vi "nanocal -- nuclear schottky fit V4.vi"() -> ()   [LabVIEW 2020]
uses:
  filename-pattern.ctl
  show-win- control.ctl
  cursor winow.ctl
  nanocal_data_read_format.ctl
  nanocal-goodness-weighting-strategy.ctl
  <vilib>/gmath/NumericalOptimization/stopping criteria.ctl
  3-lorentzian-parameters.ctl
  3-lorentzian-heat-response action.ctl
  nameformattingitem.ctl
  nanocal_side_selector.ctl
  filename-action.ctl
  cursor window action.ctl
  cursor action.ctl
  publisher action.ctl
  mathematica string map action.ctl
  array action.ctl
  cursor sate.ctl
  <vilib>/gmath/NumericalOptimization/objective function data.ctl
  3-lorentzian-parameters -- action.ctl
  <vilib>/Utility/miscctls.llb/LVMapReplaceAction.ctl
  file -- read-write control.ctl
  array -- freq-voltage transformations action.ctl
  nanocal_raw_file_manage_action_V1.ctl
  KM_file -- read-write control.ctl
  2Dwindow.ctl
  replace cursor action stack.vi
  Q -- range multiplier -- real -- V2.vi
  Q - not nan and gtr than zero - Real.vi
  Q - not nan -- real.vi
  Q -- check range -- i -- real.vi
  array - smart min max.vi
  3-lorentzian-heat-response -- analytic derivatives -- grad and curvature -- V4.vi
  <vilib>/Analysis/baseanly.llb/A x B.vi
  <vilib>/Analysis/baseanly.llb/Real A x B.vi
  <vilib>/Analysis/_algsub.llb/Matrix Norm.vi
  <vilib>/Analysis/_algsub.llb/Real Matrix Norm.vi
  3-lorentzian-heat-response -- V4.vi/142dd4c5-f9ed-c64b-bc14-a88e3e2c450a.vi
  array -- freq-voltage transformations.vi/05c44075-957c-bc42-b6fa-2799d0bc0485.vi
  tale of three indices.vi
  filter -- window span logic.vi
  linear interp iiii- complex - z-omega - divide.vi
  linear interpolation iiii- complex.vi
  containing bix.vi
  3-lorentzian-heat-response.vi/142dd4c5-f9ed-c64b-bc14-a88e3e2c450a.vi
  <vilib>/Array/Sort 2D Array - Pop Stack.vi
  <vilib>/Array/Sort 2D Array - Push Stack.vi
  array -- freq-voltage transformations.vi/05c44075-957c-bc42-b6fa-2799d0bc0485.vi/5dd0d2be-718e-c148-b8fa-e083cdba2843.vi
  array -- freq-voltage transformations.vi/05c44075-957c-bc42-b6fa-2799d0bc0485.vi/095795a0-771d-c341-9fed-d90d2e44c51c.vi
  command stack.vi
  tale of three indices -- check state.vi
  Q -- check range -- i -- integer.vi
  linear interp iiii- complex - z-omega.vi
  line -- complex.vi
  Q - not nan -- integer.vi
  <vilib>/Analysis/baseanly.llb/Complex A x B.vi
  <vilib>/Analysis/polynomials.llb/Multiply Polynomials.vi
  <vilib>/Analysis/polynomials.llb/Multiply Polynomials (DBL).vi
  <vilib>/Analysis/polynomials.llb/Polynomial Roots.vi
  <vilib>/Analysis/polynomials.llb/Polynomial Roots (DBL).vi
  array -- 3-finitediff.vi
  <vilib>/Analysis/Matrix/Numeric/Conversions/Array To Matrix.vi
  <vilib>/Analysis/Matrix/Numeric/Conversions/Array To Matrix - RA2.vi
  <vilib>/Analysis/baseanly.llb/Inverse Matrix.vi
  <vilib>/Analysis/baseanly.llb/Real Inverse Matrix.vi
  <vilib>/Analysis/Matrix/Numeric/Conversions/Array To Matrix - RA.vi
  <vilib>/Analysis/Matrix/Numeric/Conversions/Matrix To Array.vi
  <vilib>/Analysis/Matrix/Numeric/Conversions/Matrix To Array - RM.vi
  <vilib>/gmath/NumericalOptimization/Quasi Newton.vi
  <vilib>/Comparison/Less/Less Functor/Less Functor.lvclass
  <vilib>/gmath/NI_Gmath.lvlib
panel:
  in  "tab 8":enum32{"main", "Page 2"}(tab)
  in  "sweeper panel":T1(tab)
  out "Plot: sweep window":cluster{"Freq out (Hz)":dbl[], dbl[]}[](graph)
  in  "scale gauge: Plot: complex plane":dbl(slide)=2218235261.0985317 min=0.0 max=0.3 step=1e-06 scale=1000000.0..100000000000.0 scale format="%#_3p"
  in  "cspan":dbl=0.003 format="%#_13g"
  in  "cursor window":T2={"left"=20184.313682072192, "right "=24669.14654231211, "center"=22426.730112192152, "window"=4484.832860239923, "cursors"=[0, 1, 2], "relative"=0, "absolute"=0, "fixed vertical offset"=0.0, "vertical offset"=0.0, "skew"=0.0, "default window frac"=0.1, "kind"=enum."symmetric", "skew.left"=0.5, "skew.right"=0.5, "Plot ref"=refnum, "wing order"=enum."forw"}
  in  "win":T3={"cen (Hz)"=23772.179970264126, "win (Hz)"=4484.832860239923, "left (Hz)"=21529.763540144166, "right (Hz)"=26014.596400384085}
  in  ":sweep is ON":bool
  in  "stopping criteria":T4={"function tolerance"=1e-06, "parameter tolerance"=1e-06, "max iterations"=100, "max function calls"=1000, "gradient tolerance"=1e-06, "max time (sec)"=-1.0}
  in  "uco! :u":bool
  out "cursor x selector":map{T5, dbl}(c390)={enum."T (K)"=0.308, enum."B (T)"=5.0, enum."θ (deg)"=90.0}
  in  "save data":enum32{"save/read"}(tab)
  in  "Save to file :s":bool
  in  "Freq sweep name template":T6={"prefix"="RuCl3-rod", "group"="f"}
  in  "Save folder":path=path "/opt/data"
  in  "freq sweep file name":string="f013_RuCl3-rod_082821.dat"
  in  "newton control 2":T7(tab)
  in  "newton control":enum32{"Page 1"}(tab)
  in  "factor":dbl(slide)=0.0002571190773967461 scale=1e-06..1.0 scale format="%#_3p"
  in  "# steps":i32=150
  out "goodness":dbl=0.9117783129874744 format="%#_3p"
  in  "tab 4":enum32{"Page 1"}(tab)
  in  "pause!":bool
  in  "go!":bool
  in  "weighting":T8=enum."dω √(|dz/dω|)"
  in  "newton action":T9=enum."onlygrads"
  out "logarithmic derivatives":dbl[](array[numeric])=[1.000271982197808, -0.003162692351510814, -0.3377538064034027, -0.041334105920099534, -0.26981555641724986, -3.2659153548635063] format="%#_3g"
  in  "what":cluster{"scaling":dbl, "what":T5}[](array[cluster])=[{"scaling"=1.0, "what"=enum."ζ"}, {"scaling"=1.0, "what"=enum."τ1"}, {"scaling"=1.0, "what"=enum."τS"}, {"scaling"=1.0, "what"=enum."τN"}, {"scaling"=1.0, "what"=enum."τC"}, {"scaling"=1.0, "what"=enum."κ0"}]
  in  "parameters":enum32{"Page 1"}(tab)
  in  "τC":dbl(slide)=0.001074349295 min=0.0 max=0.3 step=1e-06 scale=0.0001..10.0 scale format="%#_3p"
  in  "τN":dbl(slide)=0.015552411517 min=0.0 max=0.3 step=1e-06 scale=1e-06..1000.0 scale format="%#_3p"
  in  "τS":dbl(slide)=0.109874895668 min=0.0 max=0.3 step=1e-06 scale=0.0001..10.0 scale format="%#_3p"
  in  "ζ":dbl(slide)=0.269210160049 min=0.0 max=0.3 step=1e-06 scale=1e-05..1000.0 scale format="%#_3p"
  in  "T1":dbl(slide)=0.027533256233 min=0.0 max=0.3 step=1e-06 scale=0.0001..1000.0 scale format="%#_3p"
  in  "κ0":dbl(slide)=7.32e-10 min=0.0 max=0.3 step=1e-12 scale=1e-10..1e-06 scale format="%#_3p"
  in  "newton pause":bool
  in  "plots":T10(tab)
  out "Plot:  colors":cluster{"Freq out (Hz)":dbl[], dbl[]}[](graph)=[{"Freq out (Hz)"=[0.122, 0.148, 0.168, 0.197, 0.25, 0.3, 0.36, 0.43, 0.53, 0.63, 0.83, 1.13, 1.25, 1.31, 1.39, 1.52, 1.9, 3.11, 5.75], [0.444097524539, 0.358674724692, 0.28903399494, 0.217996441376, 0.126932147164, 0.087249653273, 0.062586766538, 0.047320664202, 0.03714789601, 0.028995432115, 0.021158107821, 0.017074092265, 0.016160769926, 0.016101273075, 0.016250541117, 0.017157539727, 0.016425367394, 0.015227705493, 0.018884017265]}, {"Freq out (Hz)"=[0.122, 0.148, 0.168, 0.197, 0.25, 0.3, 0.36, 0.43, 0.53, 0.63, 0.83, 1.13, 1.25, 1.31, 1.39, 1.52, 1.9, 3.11, 5.75], [0.128858676931, 0.106557394659, 0.085284172773, 0.079837328848, 0.058068643235, 0.047168507247, 0.048322657274, 0.050730770684, 0.047226564206, 0.046559455187, 0.04718187766, 0.047215899415, 0.047360928893, 0.047373144247, 0.047393343666, 0.046379456311, 0.039829137916, 0.038797003927, 0.038756536887]}, {"Freq out (Hz)"=[0.122, 0.148, 0.168, 0.197, 0.25, 0.3, 0.36, 0.43, 0.53, 0.63, 0.83, 1.13, 1.25, 1.31, 1.39, 1.52, 1.9, 3.11, 5.75], [0.109017650637, 0.062757387956, 0.050519531224, 0.035140385542, 0.026925290066, 0.024336865487, 0.023582446152, 0.023716512211, 0.024619467421, 0.026126949833, 0.030519366684, 0.039490388664, 0.041725389227, 0.040453117489, 0.029998719281, 0.015264158508, 0.010121167967, 0.007286355621, 0.005123025136]}, {"Freq out (Hz)"=[0.122, 0.148, 0.168, 0.197, 0.25, 0.3, 0.36, 0.43, 0.53, 0.63, 0.83, 1.13, 1.25, 1.31, 1.39, 1.52, 1.9, 3.11, 5.75], [0.152310736136, 0.083491977845, 0.055850802998, 0.027062270101, 0.010981117446, 0.005605961335, 0.003596780616, 0.00220007216, 0.001310789285, 0.000676599034, 0.00025787841, 0.000122819272, 7.671595e-05, 7.667848e-05, 7.6850447e-05, 5.7006071e-05, 3.3814494e-05, 1.3994204e-05, 4.793994e-06]}, {"Freq out (Hz)"=[0.122, 0.148, 0.168, 0.197, 0.25, 0.3, 0.36, 0.43, 0.53, 0.63, 0.83, 1.13, 1.25, 1.31, 1.39, 1.52, 1.9, 3.11, 5.75], [0.001225116605, 0.001111110425, 0.001015487958, 0.001091238478, 0.001219952265, 0.001526895316, 0.001965770478, 0.002249629457, 0.002565709752, 0.003300199116, 0.004211881541, 0.004722965607, 0.004871049589, 0.005036745304, 0.004810494325, 0.004702188691, 0.004533563026, 0.003959851165, 0.002621800478]}]
  out "state of all selectors":map{T5, map{bool, dbl}}(c390)={enum."T (K)"={TRUE=0.179}, enum."B (T)"={FALSE=8.0}, enum."θ (deg)"={FALSE=0.0}, enum."side (S|R)"={FALSE=4000.0}, enum."change (B|T)"={FALSE=1.0}}
  out "state of all selectors string":string="__8.0T__0.0deg__4000side_"
  out "new selector names":map{T5, map{T11, string}}(c390)={enum."ζ"={enum."name"="ζ", enum."nameL"="zeta", enum."units"="sec", enum."prec"="%_4p"}, enum."τ1"={enum."name"="τ1", enum."nameL"="tau1", enum."units"="sec", enum."prec"="%_4p"}, enum."τS"={enum."name"="τS", enum."nameL"="tauS", enum."units"="sec", enum."prec"="%_4p"}, enum."τN"={enum."name"="τN", enum."nameL"="tauN", enum."units"="sec", enum."prec"="%_4p"}, enum."τC"={enum."name"="τC", enum."nameL"="tauC", enum."units"="sec", enum."prec"="%_4p"}, enum."κ0"={enum."name"="κ0", enum."nameL"="kappa0", enum."units"="WperK", enum."prec"="%_5p"}, enum."T (K)"={enum."name"="T", enum."nameL"="T", enum."units"="K", enum."prec"="%_4p"}, enum."B (T)"={enum."name"="B", enum."nameL"="B", enum."units"="T", enum."prec"="%_2p"}, enum."θ (deg)"={enum."name"="θ", enum."nameL"="theta", enum."units"="deg", enum."prec"="%_2p"}, enum."side (S|R)"={enum."name"="side", enum."nameL"="side", enum."units"="side", enum."prec"="%d"}}
  in  "cursor index map":map{T5, i32}(c390)={enum."ζ"=0, enum."τ1"=1, enum."τS"=2, enum."τN"=3, enum."τC"=4, enum."κ0"=5, enum."m1"=6, enum."m2"=7, enum."m3"=8}
  out "all full filenames":map{string, path}(c390)
  in  "strings stuff tab":T12(tab)
  in  "string IN":string="  \"IDS0158_210310_RAW_cal__ref_\" ->   <| \"ζ\"->  0.331549170129  , \"τ1\"-> 0.031957261989  , \"τS\"-> 0.245155954508  , \"τN\"-> 0.327332604975  , \"τC\"-> 0.001044440547  , \"κ0\"-> 0.000000000511  , \"mm1\"-> 0.000000000000  , \"mm2\"-> 0.000000000000  , \"mm3\"-> 0.000000000000  , \"T\"->  0.140000000000  , \"B\"-> 12.000000000000  , \"θ\"-> 0.000000000000  |>   , \n\"IDS0158_210310_RAW_cal__sam_\" ->   <| \"ζ\"->  0.286336668596  , \"τ1\"-> 0.037477267671  , \"τS\"-> 0.354459287884  , \"τN\"-> 0.444916383639  , \"τC\"-> 0.001225600579  , \"κ0\"-> 0.000000000596  , \"mm1\"-> 0.000000000000  , \"mm2\"-> 0.000000000000  , \"mm3\"-> 0.000000000000  , \"T\"->  0.140000000000  , \"B\"-> 12.000000000000  , \"θ\"-> 0.000000000000  |>   , \n\"IDS0159_210310_RAW_cal__ref_\" ->   <| \"ζ\"->  0.269623663752  , \"τ1\"-> 0.029946823009  , \"τS\"-> 0.193020268264  , \"τN\"-> 0.181925572107  , \"τC\"-> 0.001029221853  , \"κ0\"-> 0.000000000645  , \"mm1\"-> 0.000000000000  , \"mm2\"-> 0.000000000000  , \"mm3\"-> 0.000000000000  , \"T\"->  0.170000000000  , \"B\"-> 12.000000000000  , \"θ\"-> 0.000000000000  |>   , \n\"IDS0159_210310_RAW_cal__sam_\" ->   <| \"ζ\"->  0.219100303741  , \"τ1\"-> 0.028643012604  , \"τS\"-> 0.279362928811  , \"τN\"-> 0.246156444058  , \"τC\"-> 0.001272401549  , \"κ0\"-> 0.000000000760  , \"mm1\"-> 0.000000000000  , \"mm2\"-> 0.000000000000  , \"mm3\"-> 0.000000000000  , \"T\"->  0.170000000000  , \"B\"-> 12.000000000000  , \"θ\"-> 0.000000000000  |>   , \n\"IDS0160_210310_RAW_cal__ref_\" ->   <| \"ζ\"->  0.207047266456  , \"τ1\"-> 0.027475093360  , \"τS\"-> 0.117497913331  , \"τN\"-> 0.102020652890  , \"τC\"-> 0.000950950989  , \"κ0\"-> 0.000000000918  , \"mm1\"-> 0.000000000000  , \"mm2\"-> 0.000000000000  , \"mm3\"-> 0.000000000000  , \"T\"->  0.200000000000  , \"B\"-> 12.000000000000  , \"θ\"-> 0.000000000000  |>   , \n\"IDS0160_210310_RAW_cal__sam_\" ->   <| \"ζ\"->  0.170488637524  , \"τ1\"-> 0.029234231120  , \"τS\"-> 0.149095458227  , \"τN\"-> 0.151792620275  , \"τC\"-> 0.001113424175  , \"κ0\"-> 0.000000001042  , \"mm1\"-> 0.000000000000  , \"mm2\"-> 0.000000000000  , \"mm3\"-> 0.000000000000  , \"T\"->  0.200000000000  , \"B\"-> 12.000000000000  , \"θ\"-> 0.000000000000  |>   , \n\"IDS0161_210310_RAW_cal__ref_\" ->   <| \"ζ\"->  0.165418845287  , \"τ1\"-> 0.025256902580  , \"τS\"-> 0.095232124148  , \"τN\"-> 0.068477414693  , \"τC\"-> 0.001100413424  , \"κ0\"-> 0.000000001058  , \"mm1\"-> 0.000000000000  , \"mm2\"-> 0.000000000000  , \"mm3\"-> 0.000000000000  , \"T\"->  0.220000000000  , \"B\"-> 12.000000000000  , \"θ\"-> 0.000000000000  |>   , \n\"IDS0161_210310_RAW_cal__sam_\" ->   <| \"ζ\"->  0.130531197151  , \"τ1\"-> 0.025704482770  , \"τS\"-> 0.129606657196  , \"τN\"-> 0.091602369165  , \"τC\"-> 0.001441379995  , \"κ0\"-> 0.000000001211  , \"mm1\"-> 0.000000000000  , \"mm2\"-> 0.000000000000  , \"mm3\"-> 0.000000000000  , \"T\"->  0.220000000000  , \"B\"-> 12.000000000000  , \"θ\"-> 0.000000000000  |>   , \n\"IDS0162_210310_RAW_cal__ref_\" ->   <| \"ζ\"->  0.094488415983  , \"τ1\"-> 0.023440091411  , \"τS\"-> 0.070629137621  , \"τN\"-> 0.023695223047  , \"τC\"-> 0.001462465509  , \"κ0\"-> 0.000000001371  , \"mm1\"-> 0.000000000000  , \"mm2\"-> 0.000000000000  , \"mm3\"-> 0.000000000000  , \"T\"->  0.280000000000  , \"B\"-> 12.000000000000  , \"θ\"-> 0.000000000000  |>   , \n\"IDS0162_210310_RAW_cal__sam_\" ->   <| \"ζ\"->  0.078258046754  , \"τ1\"-> 0.028009840731  , \"τS\"-> 0.092122038762  , \"τN\"-> 0.030129595899  , \"τC\"-> 0.001641062244  , \"κ0\"-> 0.000000001543  , \"mm1\"-> 0.000000000000  , \"mm2\"-> 0.000000000000  , \"mm3\"-> 0.000000000000  , \"T\"->  0.280000000000  , \"B\"-> 12.000000000000  , \"θ\"-> 0.000000000000  |>   , \n\"IDS0163_210310_RAW_cal__ref_\" ->   <| \"ζ\"->  0.066045279838  , \"τ1\"-> 0.021690723483  , \"τS\"-> 0.054398710223  , \"τN\"-> 0.012159058060  , \"τC\"-> 0.001677829713  , \"κ0\"-> 0.000000001745  , \"mm1\"-> 0.000000000000  , \"mm2\"-> 0.000000000000  , \"mm3\"-> 0.000000000000  , \"T\"->  0.330000000000  , \"B\"-> 12.000000000000  , \"θ\"-> 0.000000000000  |>   , \n\"IDS0163_210310_RAW_cal__sam_\" ->   <| \"ζ\"->  0.054088186012  , \"τ1\"-> 0.023838802615  , \"τS\"-> 0.069079396629  , \"τN\"-> 0.016435267456  , \"τC\"-> 0.002025071743  , \"κ0\"-> 0.000000001955  , \"mm1\"-> 0.000000000000  , \"mm2\"-> 0.000000000000  , \"mm3\"-> 0.000000000000  , \"T\"->  0.330000000000  , \"B\"-> 12.000000000000  , \"θ\"-> 0.000000000000  |>   , \n\"IDS0164_210310_RAW_cal__ref_\" ->   <| \"ζ\"->  0.046429657722  , \"τ1\"-> 0.021005913305  , \"τS\"-> 0.044250298502  , \"τN\"-> 0.006399419767  , \"τC\"-> 0.002349605146  , \"κ0\"-> 0.000000002166  , \"mm1\"-> 0.000000000000  , \"mm2\"-> 0.000000000000  , \"mm3\"-> 0.000000000000  , \"T\"->  0.400000000000  , \"B\"-> 12.000000000000  , \"θ\"-> 0.000000000000  |>   , \n\"IDS0164_210310_RAW_cal__sam_\" ->   <| \"ζ\"->  0.039314966212  , \"τ1\"-> 0.020712803909  , \"τS\"-> 0.055413767550  , \"τN\"-> 0.008474403424  , \"τC\"-> 0.002674063387  , \"κ0\"-> 0.000000002415  , \"mm1\"-> 0.000000000000  , \"mm2\"-> 0.000000000000  , \"mm3\"-> 0.000000000000  , \"T\"->  0.400000000000  , \"B\"-> 12.000000000000  , \"θ\"-> 0.000000000000  |>   , \n\"IDS0165_210310_RAW_cal__ref_\" ->   <| \"ζ\"->  0.033449822896  , \"τ1\"-> 0.018946770596  , \"τS\"-> 0.035864277160  , \"τN\"-> 0.004007639534  , \"τC\"-> 0.003128970761  , \"κ0\"-> 0.000000002686  , \"mm1\"-> 0.000000000000  , \"mm2\"-> 0.000000000000  , \"mm3\"-> 0.000000000000  , \"T\"->  0.480000000000  , \"B\"-> 12.000000000000  , \"θ\"-> 0.000000000000  |>   , \n\"IDS0165_210310_RAW_cal__sam_\" ->   <| \"ζ\"->  0.031945976845  , \"τ1\"-> 0.019000922826  , \"τS\"-> 0.045624146388  , \"τN\"-> 0.005314716063  , \"τC\"-> 0.002488383471  , \"κ0\"-> 0.000000002954  , \"mm1\"-> 0.000000000000  , \"mm2\"-> 0.000000000000  , \"mm3\"-> 0.000000000000  , \"T\"->  0.480000000000  , \"B\"-> 12.000000000000  , \"θ\"-> 0.000000000000  |>   , \n\"IDS0166_210310_RAW_cal__ref_\" ->   <| \"ζ\"->  0.026131121682  , \"τ1\"-> 0.018837612836  , \"τS\"-> 0.029051745056  , \"τN\"-> 0.002477027845  , \"τC\"-> 0.003638595201  , \"κ0\"-> 0.000000003369  , \"mm1\"-> 0.000000000000  , \"mm2\"-> 0.000000000000  , \"mm3\"-> 0.000000000000  , \"T\"->  0.580000000000  , \"B\"-> 12.000000000000  , \"θ\"-> 0.000000000000  |>   , \n\"IDS0166_210310_RAW_cal__sam_\" ->   <| \"ζ\"->  0.023031239946  , \"τ1\"-> 0.018268814012  , \"τS\"-> 0.037269400776  , \"τN\"-> 0.002696792890  , \"τC\"-> 0.003257395394  , \"κ0\"-> 0.000000003720  , \"mm1\"-> 0.000000000000  , \"mm2\"-> 0.000000000000  , \"mm3\"-> 0.000000000000  , \"T\"->  0.580000000000  , \"B\"-> 12.000000000000  , \"θ\"-> 0.000000000000  |>   , \n\"IDS0167_210310_RAW_cal__ref_\" ->   <| \"ζ\"->  0.026557278794  , \"τ1\"-> 0.016933945977  , \"τS\"-> 0.022881111855  , \"τN\"-> 0.001392473895  , \"τC\"-> 0.004119437148  , \"κ0\"-> 0.000000003981  , \"mm1\"-> 0.000000000000  , \"mm2\"-> 0.000000000000  , \"mm3\"-> 0.000000000000  , \"T\"->  0.680000000000  , \"B\"-> 12.000000000000  , \"θ\"-> 0.000000000000  |>   , \n\"IDS0167_210310_RAW_cal__sam_\" ->   <| \"ζ\"->  0.019920170845  , \"τ1\"-> 0.016368892412  , \"τS\"-> 0.030579536580  , \"τN\"-> 0.001736017565  , \"τC\"-> 0.004971418152  , \"κ0\"-> 0.000000004410  , \"mm1\"-> 0.000000000000  , \"mm2\"-> 0.000000000000  , \"mm3\"-> 0.000000000000  , \"T\"->  0.680000000000  , \"B\"-> 12.000000000000  , \"θ\"-> 0.000000000000  |>   , \n\"IDS0168_210310_RAW_cal__ref_\" ->   <| \"ζ\"->  0.022041296958  , \"τ1\"-> 0.014045615335  , \"τS\"-> 0.018889590451  , \"τN\"-> 0.000813465770  , \"τC\"-> 0.004122617309  , \"κ0\"-> 0.000000005540  , \"mm1\"-> 0.000000000000  , \"mm2\"-> 0.000000000000  , \"mm3\"-> 0.000000000000  , \"T\"->  0.910000000000  , \"B\"-> 12.000000000000  , \"θ\"-> 0.000000000000  |>   , \n\"IDS0168_210310_RAW_cal__sam_\" ->   <| \"ζ\"->  0.017558473054  , \"τ1\"-> 0.014545104284  , \"τS\"-> 0.022979681288  , \"τN\"-> 0.000840829385  , \"τC\"-> 0.005228030240  , \"κ0\"-> 0.000000006068  , \"mm1\"-> 0.000000000000  , \"mm2\"-> 0.000000000000  , \"mm3\"-> 0.000000000000  , \"T\"->  0.910000000000  , \"B\"-> 12.000000000000  , \"θ\"-> 0.000000000000  |>   , \n\"IDS0169_210310_RAW_cal__ref_\" ->   <| \"ζ\"->  0.021090283514  , \"τ1\"-> 0.013945744068  , \"τS\"-> 0.014386606899  , \"τN\"-> 0.000345175874  , \"τC\"-> 0.004902956629  , \"κ0\"-> 0.000000007742  , \"mm1\"-> 0.000000000000  , \"mm2\"-> 0.000000000000  , \"mm3\"-> 0.000000000000  , \"T\"->  1.230000000000  , \"B\"-> 12.000000000000  , \"θ\"-> 0.000000000000  |>   , \n\"IDS0169_210310_RAW_cal__sam_\" ->   <| \"ζ\"->  0.011916480594  , \"τ1\"-> 0.012551282481  , \"τS\"-> 0.018233218660  , \"τN\"-> 0.000345702746  , \"τC\"-> 0.004699451527  , \"κ0\"-> 0.000000008451  , \"mm1\"-> 0.000000000000  , \"mm2\"-> 0.000000000000  , \"mm3\"-> 0.000000000000  , \"T\"->  1.230000000000  , \"B\"-> 12.000000000000  , \"θ\"-> 0.000000000000  |>   , \n\"IDS0170_210310_RAW_cal__ref_\" ->   <| \"ζ\"->  0.021449250230  , \"τ1\"-> 0.014564522147  , \"τS\"-> 0.008878867204  , \"τN\"-> 0.000064984242  , \"τC\"-> 0.006207353748  , \"κ0\"-> 0.000000012530  , \"mm1\"-> 0.000000000000  , \"mm2\"-> 0.000000000000  , \"mm3\"-> 0.000000000000  , \"T\"->  1.970000000000  , \"B\"-> 12.000000000000  , \"θ\"-> 0.000000000000  |>   , \n\"IDS0170_210310_RAW_cal__sam_\" ->   <| \"ζ\"->  0.012831327568  , \"τ1\"-> 0.013315909415  , \"τS\"-> 0.012590836847  , \"τN\"-> 0.000065003013  , \"τC\"-> 0.005276356243  , \"κ0\"-> 0.000000013610  , \"mm1\"-> 0.000000000000  , \"mm2\"-> 0.000000000000  , \"mm3\"-> 0.000000000000  , \"T\"->  1.970000000000  , \"B\"-> 12.000000000000  , \"θ\"-> 0.000000000000  |>   , \n\"IDS0171_210310_RAW_cal__ref_\" ->   <| \"ζ\"->  0.024633693577  , \"τ1\"-> 0.014940694735  , \"τS\"-> 0.006137734482  , \"τN\"-> 0.000014567254  , \"τC\"-> 0.005080683927  , \"κ0\"-> 0.000000022488  , \"mm1\"-> 0.000000000000  , \"mm2\"-> 0.000000000000  , \"mm3\"-> 0.000000000000  , \"T\"->  3.190000000000  , \"B\"-> 12.000000000000  , \"θ\"-> 0.000000000000  |>   , \n\"IDS0171_210310_RAW_cal__sam_\" ->   <| \"ζ\"->  0.019774146838  , \"τ1\"-> 0.013257273421  , \"τS\"-> 0.007064131508  , \"τN\"-> 0.000028000819  , \"τC\"-> 0.006942241845  , \"κ0\"-> 0.000000023477  , \"mm1\"-> 0.000000000000  , \"mm2\"-> 0.000000000000  , \"mm3\"-> 0.000000000000  , \"T\"->  3.190000000000  , \"B\"-> 12.000000000000  , \"θ\"-> 0.000000000000  |>   , \n\"IDS0172_210310_RAW_cal__ref_\" ->   <| \"ζ\"->  0.027835388666  , \"τ1\"-> 0.013976390421  , \"τS\"-> 0.003539188638  , \"τN\"-> 0.000003774856  , \"τC\"-> 0.004420299329  , \"κ0\"-> 0.000000055482  , \"mm1\"-> 0.000000000000  , \"mm2\"-> 0.000000000000  , \"mm3\"-> 0.000000000000  , \"T\"->  5.800000000000  , \"B\"-> 12.000000000000  , \"θ\"-> 0.000000000000  |>   , \n\"IDS0172_210310_RAW_cal__sam_\" ->   <| \"ζ\"->  0.029251354442  , \"τ1\"-> 0.014634751206  , \"τS\"-> 0.003873958746  , \"τN\"-> 0.000007000487  , \"τC\"-> 0.006827504775  , \"κ0\"-> 0.000000056438  , \"mm1\"-> 0.000000000000  , \"mm2\"-> 0.000000000000  , \"mm3\"-> 0.000000000000  , \"T\"->  5.800000000000  , \"B\"-> 12.000000000000  , \"θ\"-> 0.000000000000  |>   , \n\"IDS0181_210310_RAW_cal__ref_\" ->   <| \"ζ\"->  0.194847779603  , \"τ1\"-> 0.071300022200  , \"τS\"-> 0.034370433557  , \"τN\"-> 0.119698958932  , \"τC\"-> 0.001245041457  , \"κ0\"-> 0.000000000909  , \"mm1\"-> 0.000000000000  , \"mm2\"-> 0.000000000000  , \"mm3\"-> 0.000000000000  , \"T\"->  0.179000000000  , \"B\"-> 12.000000000000  , \"θ\"-> 90.000000000000  |>   , \n\"IDS0181_210310_RAW_cal__sam_\" ->   <| \"ζ\"->  0.161975781729  , \"τ1\"-> 0.073089805113  , \"τS\"-> 0.045018408115  , \"τN\"-> 0.161987434028  , \"τC\"-> 0.001482104484  , \"κ0\"-> 0.000000001038  , \"mm1\"-> 0.000000000000  , \"mm2\"-> 0.000000000000  , \"mm3\"-> 0.000000000000  , \"T\"->  0.179000000000  , \"B\"-> 12.000000000000  , \"θ\"-> 90.000000000000  |>   , \n\"IDS0183_210310_RAW_cal__ref_\" ->   <| \"ζ\"->  0.368639553991  , \"τ1\"-> 0.116941860160  , \"τS\"-> 0.051705641175  , \"τN\"-> 0.670097053448  , \"τC\"-> 0.001215131262  , \"κ0\"-> 0.000000000441  , \"mm1\"-> 0.000000000000  , \"mm2\"-> 0.000000000000  , \"mm3\"-> 0.000000000000  , \"T\"->  0.120000000000  , \"B\"-> 12.000000000000  , \"θ\"-> 90.000000000000  |>   , \n\"IDS0183_210310_RAW_cal__sam_\" ->   <| \"ζ\"->  0.300863384227  , \"τ1\"-> 0.104924004009  , \"τS\"-> 0.071070599729  , \"τN\"-> 0.992887187112  , \"τC\"-> 0.001721587800  , \"κ0\"-> 0.000000000548  , \"mm1\"-> 0.000000000000  , \"mm2\"-> 0.000000000000  , \"mm3\"-> 0.000000000000  , \"T\"->  0.120000000000  , \"B\"-> 12.000000000000  , \"θ\"-> 90.000000000000  |>   , \n\"IDS0184_210310_RAW_cal__ref_\" ->   <| \"ζ\"->  0.260731272629  , \"τ1\"-> 0.088447317905  , \"τS\"-> 0.043671964304  , \"τN\"-> 0.254005375090  , \"τC\"-> 0.001151280234  , \"κ0\"-> 0.000000000662  , \"mm1\"-> 0.000000000000  , \"mm2\"-> 0.000000000000  , \"mm3\"-> 0.000000000000  , \"T\"->  0.148000000000  , \"B\"-> 12.000000000000  , \"θ\"-> 90.000000000000  |>   , \n\"IDS0184_210310_RAW_cal__sam_\" ->   <| \"ζ\"->  0.215697702358  , \"τ1\"-> 0.095971807771  , \"τS\"-> 0.069319630290  , \"τN\"-> 0.366712218878  , \"τC\"-> 0.001526252261  , \"κ0\"-> 0.000000000784  , \"mm1\"-> 0.000000000000  , \"mm2\"-> 0.000000000000  , \"mm3\"-> 0.000000000000  , \"T\"->  0.148000000000  , \"B\"-> 12.000000000000  , \"θ\"-> 90.000000000000  |>   , \n\"IDS0185_210310_RAW_cal__ref_\" ->   <| \"ζ\"->  0.166318035375  , \"τ1\"-> 0.066119695107  , \"τS\"-> 0.031891479777  , \"τN\"-> 0.088107606578  , \"τC\"-> 0.001299933301  , \"κ0\"-> 0.000000001075  , \"mm1\"-> 0.000000000000  , \"mm2\"-> 0.000000000000  , \"mm3\"-> 0.000000000000  , \"T\"->  0.197000000000  , \"B\"-> 12.000000000000  , \"θ\"-> 90.000000000000  |>   , \n\"IDS0185_210310_RAW_cal__sam_\" ->   <| \"ζ\"->  0.139117463690  , \"τ1\"-> 0.070330410174  , \"τS\"-> 0.040829719954  , \"τN\"-> 0.122434321115  , \"τC\"-> 0.001436112939  , \"κ0\"-> 0.000000001208  , \"mm1\"-> 0.000000000000  , \"mm2\"-> 0.000000000000  , \"mm3\"-> 0.000000000000  , \"T\"->  0.197000000000  , \"B\"-> 12.000000000000  , \"θ\"-> 90.000000000000  |>   , \n\"IDS0186_210310_RAW_cal__ref_\" ->   <| \"ζ\"->  0.101265410351  , \"τ1\"-> 0.051590946451  , \"τS\"-> 0.026920044229  , \"τN\"-> 0.035536954174  , \"τC\"-> 0.001490330879  , \"κ0\"-> 0.000000001364  , \"mm1\"-> 0.000000000000  , \"mm2\"-> 0.000000000000  , \"mm3\"-> 0.000000000000  , \"T\"->  0.249000000000  , \"B\"-> 12.000000000000  , \"θ\"-> 90.000000000000  |>   , \n\"IDS0186_210310_RAW_cal__sam_\" ->   <| \"ζ\"->  0.079912790251  , \"τ1\"-> 0.053932962768  , \"τS\"-> 0.033847624645  , \"τN\"-> 0.047947649984  , \"τC\"-> 0.001828917906  , \"κ0\"-> 0.000000001546  , \"mm1\"-> 0.000000000000  , \"mm2\"-> 0.000000000000  , \"mm3\"-> 0.000000000000  , \"T\"->  0.249000000000  , \"B\"-> 12.000000000000  , \"θ\"-> 90.000000000000  |>   , \n\"IDS0187_210310_RAW_cal__ref_\" ->   <| \"ζ\"->  0.070401604603  , \"τ1\"-> 0.043684283216  , \"τS\"-> 0.023756676354  , \"τN\"-> 0.017570167589  , \"τC\"-> 0.001809460237  , \"κ0\"-> 0.000000001742  , \"mm1\"-> 0.000000000000  , \"mm2\"-> 0.000000000000  , \"mm3\"-> 0.000000000000  , \"T\"->  0.300000000000  , \"B\"-> 12.000000000000  , \"θ\"-> 90.000000000000  |>   , \n\"IDS0187_210310_RAW_cal__sam_\" ->   <| \"ζ\"->  0.057938569833  , \"τ1\"-> 0.045244527663  , \"τS\"-> 0.029709028064  , \"τN\"-> 0.023577376257  , \"τC\"-> 0.002006607539  , \"κ0\"-> 0.000000001948  , \"mm1\"-> 0.000000000000  , \"mm2\"-> 0.000000000000  , \"mm3\"-> 0.000000000000  , \"T\"->  0.300000000000  , \"B\"-> 12.000000000000  , \"θ\"-> 90.000000000000  |>   , \n\"IDS0188_210310_RAW_cal__ref_\" ->   <| \"ζ\"->  0.052039078112  , \"τ1\"-> 0.037833987996  , \"τS\"-> 0.021664376950  , \"τN\"-> 0.010364100672  , \"τC\"-> 0.002302914949  , \"κ0\"-> 0.000000002119  , \"mm1\"-> 0.000000000000  , \"mm2\"-> 0.000000000000  , \"mm3\"-> 0.000000000000  , \"T\"->  0.360000000000  , \"B\"-> 12.000000000000  , \"θ\"-> 90.000000000000  |>   , \n\"IDS0188_210310_RAW_cal__sam_\" ->   <| \"ζ\"->  0.044154556051  , \"τ1\"-> 0.038823125235  , \"τS\"-> 0.027069314930  , \"τN\"-> 0.013601990730  , \"τC\"-> 0.002287979276  , \"κ0\"-> 0.000000002359  , \"mm1\"-> 0.000000000000  , \"mm2\"-> 0.000000000000  , \"mm3\"-> 0.000000000000  , \"T\"->  0.360000000000  , \"B\"-> 12.000000000000  , \"θ\"-> 90.000000000000  |>   , \n\"IDS0189_210310_RAW_cal__ref_\" ->   <| \"ζ\"->  0.040584680050  , \"τ1\"-> 0.030359591877  , \"τS\"-> 0.019792901852  , \"τN\"-> 0.005324821183  , \"τC\"-> 0.002700986774  , \"κ0\"-> 0.000000002671  , \"mm1\"-> 0.000000000000  , \"mm2\"-> 0.000000000000  , \"mm3\"-> 0.000000000000  , \"T\"->  0.430000000000  , \"B\"-> 12.000000000000  , \"θ\"-> 90.000000000000  |>   , \n\"IDS0189_210310_RAW_cal__sam_\" ->   <| \"ζ\"->  0.032748569996  , \"τ1\"-> 0.031072007290  , \"τS\"-> 0.024343937548  , \"τN\"-> 0.006961654481  , \"τC\"-> 0.002967111565  , \"κ0\"-> 0.000000002964  , \"mm1\"-> 0.000000000000  , \"mm2\"-> 0.000000000000  , \"mm3\"-> 0.000000000000  , \"T\"->  0.430000000000  , \"B\"-> 12.000000000000  , \"θ\"-> 90.000000000000  |>   , \n\"IDS0190_210310_RAW_cal__ref_\" ->   <| \"ζ\"->  0.030700897923  , \"τ1\"-> 0.026935085078  , \"τS\"-> 0.018364864329  , \"τN\"-> 0.002898516959  , \"τC\"-> 0.003150649099  , \"κ0\"-> 0.000000003342  , \"mm1\"-> 0.000000000000  , \"mm2\"-> 0.000000000000  , \"mm3\"-> 0.000000000000  , \"T\"->  0.512000000000  , \"B\"-> 12.000000000000  , \"θ\"-> 90.000000000000  |>   , \n\"IDS0190_210310_RAW_cal__sam_\" ->   <| \"ζ\"->  0.027599263457  , \"τ1\"-> 0.026239105728  , \"τS\"-> 0.022370859308  , \"τN\"-> 0.003857632966  , \"τC\"-> 0.003499360499  , \"κ0\"-> 0.000000003681  , \"mm1\"-> 0.000000000000  , \"mm2\"-> 0.000000000000  , \"mm3\"-> 0.000000000000  , \"T\"->  0.512000000000  , \"B\"-> 12.000000000000  , \"θ\"-> 90.000000000000  |>   , \n\"IDS0191_210310_RAW_cal__ref_\" ->   <| \"ζ\"->  0.025322625458  , \"τ1\"-> 0.023401812401  , \"τS\"-> 0.017347416709  , \"τN\"-> 0.002020498851  , \"τC\"-> 0.003594259467  , \"κ0\"-> 0.000000003970  , \"mm1\"-> 0.000000000000  , \"mm2\"-> 0.000000000000  , \"mm3\"-> 0.000000000000  , \"T\"->  0.610000000000  , \"B\"-> 12.000000000000  , \"θ\"-> 90.000000000000  |>   , \n\"IDS0191_210310_RAW_cal__sam_\" ->   <| \"ζ\"->  0.020568815513  , \"τ1\"-> 0.023045965648  , \"τS\"-> 0.020791387386  , \"τN\"-> 0.002229171297  , \"τC\"-> 0.004427475438  , \"κ0\"-> 0.000000004398  , \"mm1\"-> 0.000000000000  , \"mm2\"-> 0.000000000000  , \"mm3\"-> 0.000000000000  , \"T\"->  0.610000000000  , \"B\"-> 12.000000000000  , \"θ\"-> 90.000000000000  |>   , \n\"IDS0192_210310_RAW_cal__ref_\" ->   <| \"ζ\"->  0.022100596026  , \"τ1\"-> 0.020519097823  , \"τS\"-> 0.015555141042  , \"τN\"-> 0.000889956832  , \"τC\"-> 0.004354791503  , \"κ0\"-> 0.000000005560  , \"mm1\"-> 0.000000000000  , \"mm2\"-> 0.000000000000  , \"mm3\"-> 0.000000000000  , \"T\"->  0.810000000000  , \"B\"-> 12.000000000000  , \"θ\"-> 90.000000000000  |>   , \n\"IDS0192_210310_RAW_cal__sam_\" ->   <| \"ζ\"->  0.016548170999  , \"τ1\"-> 0.020108887890  , \"τS\"-> 0.018558394948  , \"τN\"-> 0.001160732495  , \"τC\"-> 0.004746126241  , \"κ0\"-> 0.000000005882  , \"mm1\"-> 0.000000000000  , \"mm2\"-> 0.000000000000  , \"mm3\"-> 0.000000000000  , \"T\"->  0.810000000000  , \"B\"-> 12.000000000000  , \"θ\"-> 90.000000000000  |>   , \n\"IDS0193_210310_RAW_cal__ref_\" ->   <| \"ζ\"->  0.020969814378  , \"τ1\"-> 0.020016820130  , \"τS\"-> 0.013372894745  , \"τN\"-> 0.000454586591  , \"τC\"-> 0.005292751338  , \"κ0\"-> 0.000000007771  , \"mm1\"-> 0.000000000000  , \"mm2\"-> 0.000000000000  , \"mm3\"-> 0.000000000000  , \"T\"->  1.100000000000  , \"B\"-> 12.000000000000  , \"θ\"-> 90.000000000000  |>   , \n\"IDS0193_210310_RAW_cal__sam_\" ->   <| \"ζ\"->  0.014495870556  , \"τ1\"-> 0.019990087457  , \"τS\"-> 0.016832201384  , \"τN\"
